vi "niRFSysCalReader Create Interpolation Table.vi"(8 "error in":errorcluster, 11 "niRFSysCalReader Handle":T1) -> (0 "error out":errorcluster, 2 "Interpolation Table":dbl[][](array[numeric]), 3 "niRFSysCalReader Handle out":T1)   [LabVIEW 2016, in "niRFSysCalReader.lvlib"]
uses:
  niRFSysCalReader.lvlib
  _INCLUDES/niRFSysCalReader Handle.ctl
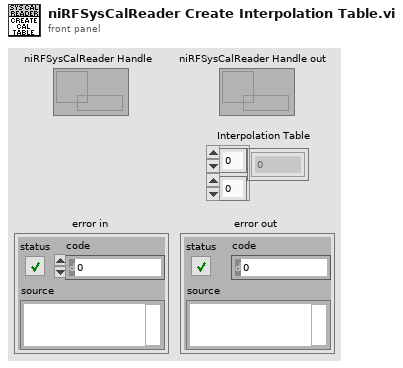
[diagram p1: front panel]
types:
  T1 = typedef "niRFSysCalReader.lvlib/niRFSysCalReader Handle.ctl" = refnum<data-value>
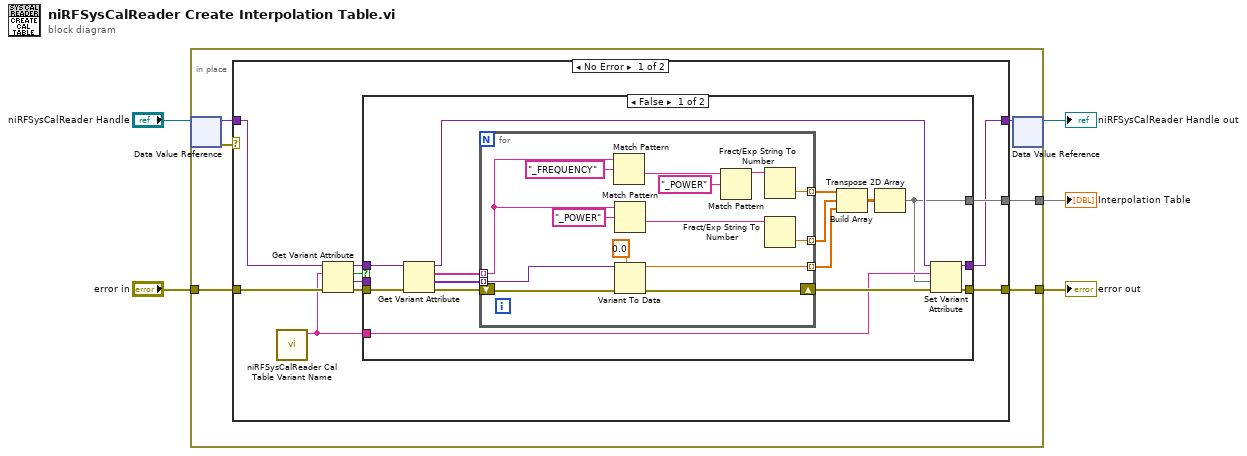
[diagram p0: block diagram]
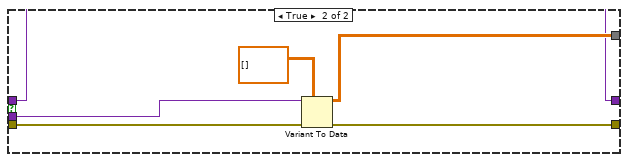
[diagram p2: hidden frame]
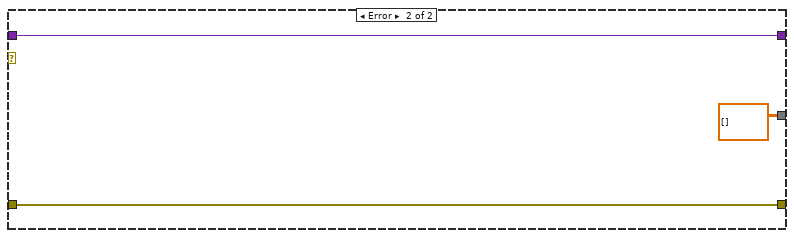
[diagram p3: hidden frame]
diagram:
  n1 = in-place {
    in-place-border: [w11] -> w5
    in-place-border: "error in" -> [w7]
    in-place-border: [w9] -> w3
    n2 = in-place-dvr #1("niRFSysCalReader Handle") -> (w8:variant, w6:errorcluster)
    n3 = case shown="No Error" w6 {
      tunnel: [w21 dbl[][] [] ("transposed array")] -> w11
      tunnel: [w20 w59] -> w10
      tunnel: [w19 w58] -> w9
      tunnel: w8 -> [w18 w59]
      tunnel: w7 -> [w17 w58]
      frame No Error {
        n4 = call "niRFSysCalReader Cal Table Variant Name.vi"() -> ("Calibration Table Name"=w15:string)  [unwired: 11 in]
        n5 = Get Variant Attribute(Variant=w18, name=w15, error in=w17) -> (duplicate Variant=w14:variant, found=w13:bool, value=w12:variant, error out=w16:errorcluster)  [unwired: 1 in]
        n6 = case shown="False" w13 {
          tunnel: [w22 w52] -> w21
          tunnel: [w28 w51] -> w20
          tunnel: [w26 w56] -> w19
          tunnel: w16 -> [w25 w54]
          tunnel: w15 -> [w24 _]
          tunnel: w14 -> [w23 w51]
          tunnel: w12 -> [_ w55]
          frame False {
            n7 = Get Variant Attribute(Variant=w23, error in=w25) -> (duplicate Variant=w29:variant, names=w36:string[], values=w35:variant[], error out=w34:errorcluster)  [unwired: 2 in]
            n8 = for {
              tunnel: [w44] -> w30 mode=indexing
              tunnel: [w43] -> w31 mode=indexing
              shift-right: [w41] -> w27
              shift-left: w34 -> [w42]
              tunnel: [w39] -> w32 mode=indexing
              tunnel: w35 -> [w38] mode=indexing
              tunnel: w36 -> [w37] mode=indexing
              n9 = Match Pattern(string=w37, regular expression="_FREQUENCY") -> (after substring=w46:string)  [unwired: 1 in, 3 out]
              n10 = Match Pattern(string=w37, regular expression="_POWER") -> (after substring=w48:string)  [unwired: 1 in, 3 out]
              n11 = Variant To Data(error in=w42, type=0.0 ("Frequency (Hz)"), Variant=w38) -> (data=w39:dbl, error out=w41:errorcluster)
              n12 = Match Pattern(string=w46, regular expression="_POWER") -> (before substring=w45:string)  [unwired: 1 in, 3 out]
              n13 = Fract/Exp String To Number(string=w45) -> (number=w44:dbl)  [unwired: 3 in, 1 out]
              n14 = Fract/Exp String To Number(string=w48) -> (number=w43:dbl)  [unwired: 3 in, 1 out]
            }
            n15 = Build Array(w30, w31, w32) -> (w33:dbl[][])
            n16 = Transpose 2D Array(2D array=w33) -> (transposed array=w22:dbl[][])
            n17 = Set Variant Attribute(Variant=w29, name=w24, value=w22, error in=w27) -> (Variant out=w28:variant, error out=w26:errorcluster)  [unwired: 1 out]
          }
          frame True {
            n18 = Variant To Data(error in=w54, type=dbl[][] [] ("transposed array"), Variant=w55) -> (data=w52:dbl[][], error out=w56:errorcluster)
          }
        }
      }
      frame Error {
      }
    }
    n19 = in-place-dvr #1(w10) -> (→"niRFSysCalReader Handle out":T1)  [unwired: 1 out]
  }
  "Interpolation Table" <- w5
  "error out" <- w3
